vi "StartSlideOut.vi"(8 "error in (no error)":errorcluster, 11 "Game in":refnum<class "Game.lvclass">) -> (0 "error out":errorcluster, 3 "Game out":refnum<class "Game.lvclass">)   [LabVIEW 2019, in "RT_Game.lvlib" / "Game.lvclass"]
uses:
  Game.lvclass
  Menu/Menu.lvclass
  Menu/States.ctl
  Game.lvclass/Game.ctl
panel:
  in  "RT_Game.lvlib:Menu.lvclass":refnum<class "Menu.lvclass">
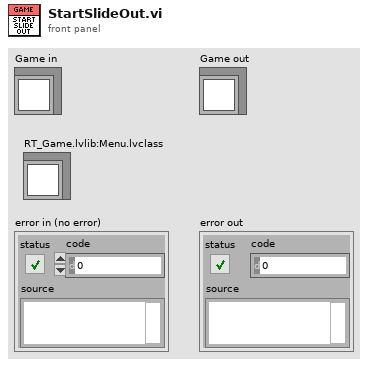
[diagram p1: front panel]
types:
  T1 = typedef "RT_Game.lvlib/Game.lvclass/States.ctl" = enum16{"Init", "Restart", "Menu", "Game", "Resume", "ToggleSingleplayer", "LoadNextGame", "ExitToMenu", "NewHighscore", "GameOver", "SlideOut"}
  T2 = typedef "RT_Game.lvlib/Game.lvclass/ScreenSide.ctl" = enum16{"up", "down", "left", "right", "none"}
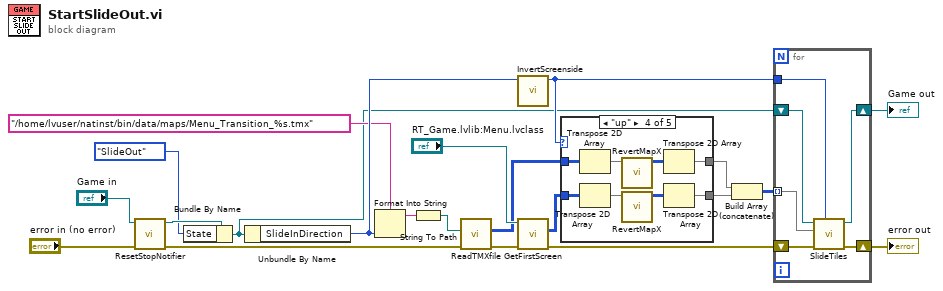
[diagram p0: block diagram]
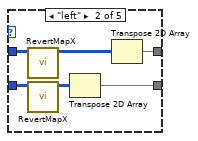
[diagram p3: hidden frame]
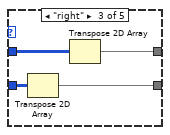
[diagram p4: hidden frame]
diagram:
  n1 = call "ResetStopNotifier.vi"("error in (no error)"="error in (no error)", "Game in"="Game in") -> ("error out"=w11:errorcluster, "Game out"=w13:refnum<class "Game.lvclass">)  [unwired: 8 in]
  n2 = Bundle By Name(cluster=w13, "State"=States."SlideOut") -> (w14:refnum<class "Game.lvclass">)
  n3 = Unbundle By Name(w14) -> ("SlideInDirection"=w17:T2)
  n4 = Format Into String(format string="/home/lvuser/natinst/bin/data/maps/Menu_Transition_%s.tmx", w17) -> (resulting string=w18:string)  [unwired: 2 in, 1 out]
  n5 = String To Path(string=w18) -> (path=w19:path)
  n6 = call "ReadTMXfile.vi"("error in (no error)"=w11, "path to tmx-file (created with Tiles2D)"=w19) -> ("error out"=w7:errorcluster, "Tilenumbers"=w3:u32[][])  [unwired: 8 in]
  n7 = call "InvertScreenside.vi"("SlideInDirection"=w17) -> ("Inverted"=w15:T2)  [unwired: 10 in]
  n8 = call-dynamic "GetFirstScreen.vi"("error in (no error)"=w7, "Menu in"="RT_Game.lvlib:Menu.lvclass") -> ("error out"=w8:errorcluster, "Array"=w10:u32[][])  [unwired: 7 in, 1 out]
  n9 = case shown="\"up\"" w15 {
    tunnel: w3 -> [w23 w28 w33 w41 w43]
    tunnel: [w23 w25 w31 w39 w43] -> w20
    tunnel: w10 -> [w22 w27 w32 w40 w42]
    tunnel: [w22 w24 w30 w38 w42] -> w21
    frame Default {
    }
    frame "left" {
      n10 = call "RevertMapX.vi"("Tilenumbers"=w28) -> ("Array"=w29:u32[][])  [unwired: 10 in]
      n11 = call "RevertMapX.vi"("Tilenumbers"=w27) -> ("Array"=w26:u32[][])  [unwired: 10 in]
      n12 = Transpose 2D Array(2D array=w26) -> (transposed array=w24:u32[][])
      n13 = Transpose 2D Array(2D array=w29) -> (transposed array=w25:u32[][])
    }
    frame "right" {
      n14 = Transpose 2D Array(2D array=w32) -> (transposed array=w30:u32[][])
      n15 = Transpose 2D Array(2D array=w33) -> (transposed array=w31:u32[][])
    }
    frame "up" {
      n16 = Transpose 2D Array(2D array=w41) -> (transposed array=w35:u32[][])
      n17 = Transpose 2D Array(2D array=w40) -> (transposed array=w34:u32[][])
      n18 = call "RevertMapX.vi"("Tilenumbers"=w35) -> ("Array"=w37:u32[][])  [unwired: 10 in]
      n19 = call "RevertMapX.vi"("Tilenumbers"=w34) -> ("Array"=w36:u32[][])  [unwired: 10 in]
      n20 = Transpose 2D Array(2D array=w37) -> (transposed array=w39:u32[][])
      n21 = Transpose 2D Array(2D array=w36) -> (transposed array=w38:u32[][])
    }
    frame "down" {
    }
  }
  n22 = Build Array (concatenate)(w20, w21) -> (w9:u32[][])
  n23 = for {
    shift-right: [w48] -> w4
    shift-left: w8 -> [w49]
    shift-right: [w46] -> w5
    shift-left: w14 -> [w47]
    tunnel: w9 -> [w45] mode=indexing
    tunnel: w15 -> [w44]
    n24 = call "SlideTiles.vi"("Side"=w44, "error in (no error)"=w49, "Tilecodes"=w45, "Game in"=w47) -> ("error out"=w48:errorcluster, "Game out"=w46:refnum<class "Game.lvclass">)  [unwired: 6 in]
  }
  "Game out" <- w5
  "error out" <- w4
